vi "GT Get Pls Pos.vi"(6 "pClock":u32, 7 "count":i16, 8 "error in (no error)":errorcluster caption="错误输入（无错误）", 9 "pValue":dbl, 10 "pulse":i16, 11 "cardNum":i16) -> (0 "error out":errorcluster caption="错误输出", 1 "pValue out":dbl, 3 "function return":i16, 4 "pClock out":u32)   [LabVIEW 2020, in "gts1.lvlib"]
doc: "GT_API GT_GetPlsPos(short cardNum,short pulse,double *pValue,short count,unsigned long *pClock);"
uses:
  gts1.lvlib
  dll/32bit/multi_card/gts.dll
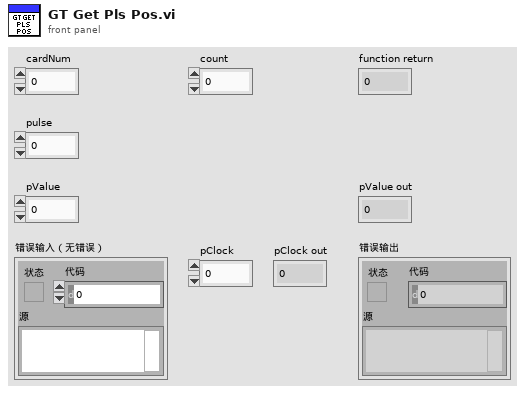
[diagram p1: front panel]
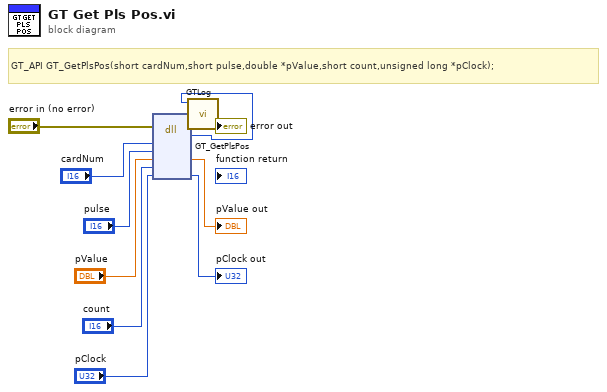
[diagram p0: block diagram]
diagram:
  # "GT_API GT_GetPlsPos(short cardNum,short pulse,double *pValue,short count,unsigned long *pClock);"
  n1 = dll-call lib="C:/1228/dll/32bit/multi_card/gts.dll" fn="GT_GetPlsPos"(error in="error in (no error)", "cardNum"="cardNum", "pulse"="pulse", "pValue"="pValue", "count"="count", "pClock"="pClock") -> (error out=w3:errorcluster, w1:i16, "pValue"=→"pValue out":dbl, "pClock"=→"pClock out":u32)  [unwired: 5 in, 1 out]
  n2 = call "GTLog.vi"("error in (no error)"=w3, "Numeric"=w1) -> ("error out"=→"error out":errorcluster)  [unwired: 9 in]
